vi "TxCommit_Core.vi"(8 "error in (no error)":errorcluster, 11 "DbConnection in":refnum<class "ORM_DBC_dotNet.lvclass">) -> (0 "error out":errorcluster, 3 "DbConnection out":refnum<class "ORM_DBC_dotNet.lvclass">)   [LabVIEW 2020, in "ORM_DBC_dotNet.lvlib" / "ORM_DBC_dotNet.lvclass"]
uses:
  ORM_DBC_dotNet.lvclass
  ORM_DBC_dotNet.lvclass/ORM_DBC_dotNet.ctl
  Read transactions.vi
  Write transactions.vi
  System.Data
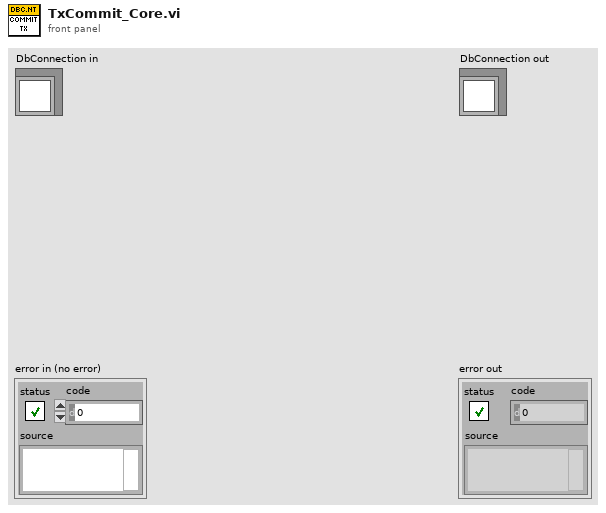
[diagram p1: front panel]
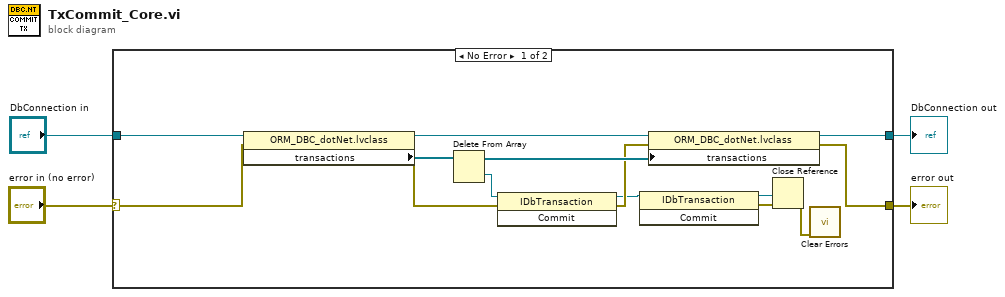
[diagram p0: block diagram]
diagram:
  n1 = case shown="No Error" "error in (no error)" {
    selector: "error in (no error)" -> [w17 w20]
    tunnel: [w16 w20] -> w3
    tunnel: [w18 w19] -> w1
    tunnel: "DbConnection in" -> [w15 w19]
    frame No Error {
      n2 = property class="ORM_DBC_dotNet.lvclass"(reference=w15, error in=w17) -> (reference out=w13:refnum<class "ORM_DBC_dotNet.lvclass">, error out=w10:errorcluster, "transactions"=w12:refnum<k24>[])
      n3 = Delete From Array(array=w12) -> (deleted portion=w14:refnum<k24>, array with subset deleted=w11:refnum<k24>[])  [unwired: 2 in]
      n4 = invoke class="IDbTransaction" method="Commit"(reference=w14, error in=w10) -> (reference out=w8:refnum<k24>, error out=w9:errorcluster)  [unwired: 1 in, 1 out]
      n5 = invoke class="IDbTransaction" method="Commit"(reference=w8) -> (reference out=w6:refnum<k24>, error out=w7:errorcluster)  [unwired: 2 in, 1 out]
      n6 = property class="ORM_DBC_dotNet.lvclass"(reference=w13, error in=w9, "transactions"=w11) -> (reference out=w18:refnum<class "ORM_DBC_dotNet.lvclass">, error out=w16:errorcluster)
      n7 = Close Reference(reference=w6, error in (no error)=w7) -> (error out=w5:errorcluster)
      n8 = call <vilib>:"Clear Errors.vi"("error in (no error)"=w5) -> ()  [unwired: 5 in, 2 out]
    }
    frame Error {
    }
  }
  "error out" <- w3
  "DbConnection out" <- w1
